vi "Set Iteration.vi"(10 "Iteration":u64=1, 11 "Timing in":refnum<class "Engine Timing.lvclass">) -> (3 "Timing out":refnum<class "Engine Timing.lvclass">)   [LabVIEW 2017, in "Data Sharing Framework Engine.lvlib" / "Engine Timing.lvclass"]
uses:
  Engine Timing.lvclass
  Engine Timing.lvclass/Engine Timing.ctl
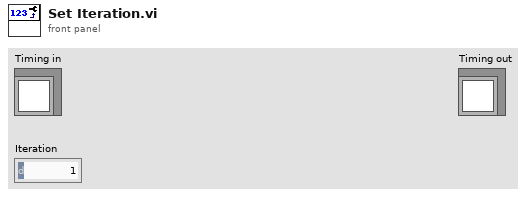
[diagram p1: front panel]
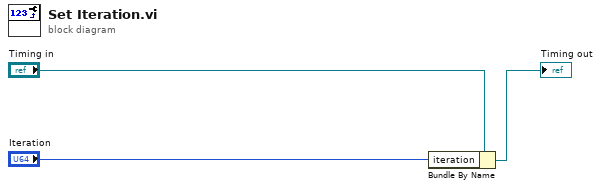
[diagram p0: block diagram]
diagram:
  n1 = Bundle By Name(cluster="Timing in", "iteration"="Iteration") -> (→"Timing out":refnum<class "Engine Timing.lvclass">)
